vi "PMX_LoadParameterSet.vi"(8 "Error in":errorcluster, 10 "ParameterSetNumber":i32, 11 "Device":refnum<k24>) -> (0 "Error out":errorcluster, 2 "Result":bool, 3 "Device":refnum<k24>)   [LabVIEW 2016]
doc: "Loads the given parameter set number. \nIf the parameter set exists and has been loaded the result is true, else false.\n\nDevice: PMX device on whicht to load the given parameter set number\nParametersetNumber: Parameter set that should be loaded (0,1,2,3...). -1 means: Load factory setup into currently active parameter set and activate it. \nResult: True, if parameter set exists and has been loaded"
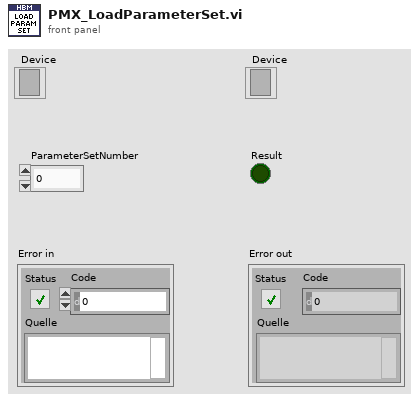
[diagram p1: front panel]
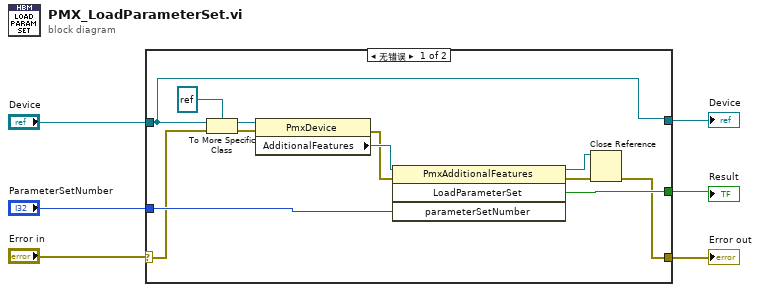
[diagram p0: block diagram]
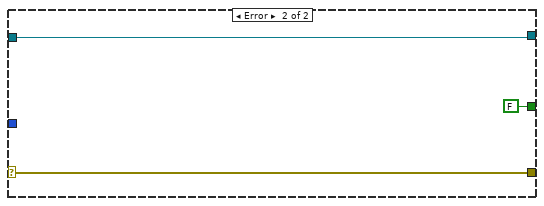
[diagram p2: hidden frame]
diagram:
  n1 = case shown="无错误" "Error in" {
    selector: "Error in" -> [w11 w21]
    tunnel: [w7 w21] -> w2
    tunnel: "ParameterSetNumber" -> [w14 _]
    tunnel: "Device" -> [w12 w19]
    tunnel: [w13 FALSE ("LoadParameterSet")] -> w4
    tunnel: [w12 w19] -> w1
    frame No Error {
      n2 = To More Specific Class(target class=refnum<k24> refnum ("Zielklasse"), reference=w12, error in=w11) -> (specific class reference=w18:refnum<k24>, error out=w15:errorcluster)
      n3 = property on="Eigenschaftsknoten" class="PmxDevice"(reference=w18, error in=w15) -> (error out=w16:errorcluster, "AdditionalFeatures"=w17:refnum<k24>)  [unwired: 1 out]
      n4 = invoke on="Methodenknoten" class="PmxAdditionalFeatures" method="LoadParameterSet"(reference=w17, error in=w16, "parameterSetNumber"=w14) -> (reference out=w8:refnum<k24>, error out=w9:errorcluster, "LoadParameterSet"=w13:bool)  [unwired: 1 in, 1 out]
      n5 = Close Reference(reference=w8, error in (no error)=w9) -> (error out=w7:errorcluster)
    }
    frame Error {
    }
  }
  "Result" <- w4
  "Error out" <- w2
  "Device" <- w1
